vi "BK Precision 8600 Series Run List File.vi"() -> ()   [LabVIEW 2018]
doc: "Exemplifies how to run a stored list (sequence) from internal memory and measuring voltage and current while sequence is initiated."
uses:
  <instrlib>/BK Precision 8600 Series/BK Precision 8600 Series.lvlib
panel:
  in  "?":bool
  out "Current":dbl
  out "Voltage":dbl format="%_6f"
  in  "List Number (1)":i32=1 min=1 max=7 format="%#_0f"
  in  "VISA resource name":refnum<visa-resource-name>
  in  "Serial Configuration":cluster{"Baud Rate":u32}={"Baud Rate"=9600} {"Baud Rate" items=["300"=300, "600"=600, "1200"=1200, "2400"=2400, "4800"=4800, "9600"=9600, "19200"=19200]}
  # "(c) 2014-2019 B&K Precision Corporation.  ALL RIGHTS RESERVED."
  # "V"
  # "A"
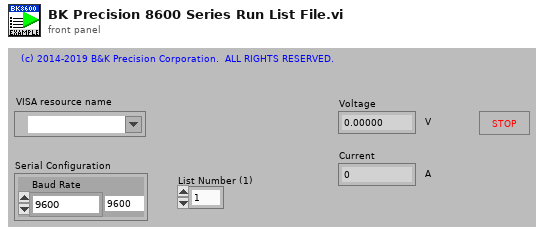
[diagram p1: front panel]
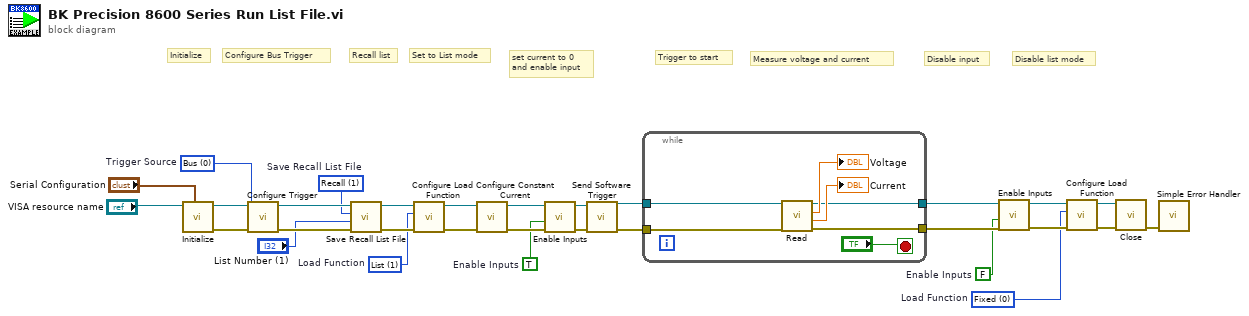
[diagram p0: block diagram]
diagram:
  w1 = u16 0 items=["Fixed", "List"]  # Load Function
  w3 = FALSE  # Enable Inputs
  w4 = TRUE  # Enable Inputs
  w2 = u16 1 items=["Fixed", "List"]  # Load Function
  w5 = u16 1 items=["Save", "Recall"]  # Save Recall List File
  w6 = u16 0 items=["Bus", "External", "Hold", "Manual", "Timed"]  # Trigger Source
  # "set current to 0\nand enable input"
  # "Measure voltage and current"
  # "Disable list mode"
  # "Set to List mode"
  # "Recall list"
  # "Configure Bus Trigger"
  # "Initialize"
  # "Trigger to start"
  # "Disable input"
  n1 = call <instrlib>:"Initialize.vi"("Serial Configuration"="Serial Configuration", "VISA resource name"="VISA resource name") -> ("error out"=w27:errorcluster, "VISA resource name out"=w28:refnum<visa-resource-name>)  [unwired: 8 in]
  n2 = call <instrlib>:"Configure Trigger.vi"("error in (no error)"=w27, "Trigger Source (0:Bus)"=w6, "VISA resource name"=w28) -> ("error out"=w24:errorcluster, "VISA resource name out"=w25:refnum<visa-resource-name>)  [unwired: 7 in]
  n3 = call <instrlib>:"Save Recall List File.vi"("error in (no error)"=w24, "List Number (1)"="List Number (1)", "Save Recall List File (0:Save)"=w5, "VISA resource name"=w25) -> ("error out"=w21:errorcluster, "VISA resource name out"=w22:refnum<visa-resource-name>)  [unwired: 6 in]
  n4 = call <instrlib>:"Configure Load Function.vi"("error in (no error)"=w21, "Load Function (0:Fixed)"=w2, "VISA resource name"=w22) -> ("error out"=w20:errorcluster, "VISA resource name out"=w19:refnum<visa-resource-name>)  [unwired: 7 in]
  n5 = call <instrlib>:"Configure Constant Current.vi"("error in (no error)"=w20, "VISA resource name"=w19) -> ("error out"=w18:errorcluster, "VISA resource name out"=w17:refnum<visa-resource-name>)  [unwired: 8 in]
  n6 = call <instrlib>:"Enable Inputs.vi"("error in (no error)"=w18, "Enable Input (F: False)"=w4, "VISA resource name"=w17) -> ("error out"=w15:errorcluster, "VISA resource name out"=w16:refnum<visa-resource-name>)  [unwired: 7 in]
  n7 = call <instrlib>:"Send Software Trigger.vi"("error in (no error)"=w15, "VISA resource name"=w16) -> ("error out"=w13:errorcluster, "VISA resource name out"=w14:refnum<visa-resource-name>)  [unwired: 8 in]
  n8 = while {
    tunnel: w14 -> [w35]
    tunnel: w13 -> [w34]
    tunnel: [w33] -> w12
    tunnel: [w32] -> w11
    stop <- "?" stop-if-true
    n9 = call <instrlib>:"Read.vi"("error in (no error)"=w34, "VISA resource name"=w35) -> ("error out"=w33:errorcluster, "Current"=→"Current":dbl, "Voltage"=→"Voltage":dbl, "VISA resource name out"=w32:refnum<visa-resource-name>)  [unwired: 6 in]
  }
  n10 = call <instrlib>:"Enable Inputs.vi"("error in (no error)"=w12, "Enable Input (F: False)"=w3, "VISA resource name"=w11) -> ("error out"=w9:errorcluster, "VISA resource name out"=w10:refnum<visa-resource-name>)  [unwired: 7 in]
  n11 = call <instrlib>:"Configure Load Function.vi"("error in (no error)"=w9, "Load Function (0:Fixed)"=w1, "VISA resource name"=w10) -> ("error out"=w7:errorcluster, "VISA resource name out"=w8:refnum<visa-resource-name>)  [unwired: 7 in]
  n12 = call <instrlib>:"Close.vi"("error in (no error)"=w7, "VISA resource name"=w8) -> ("error out"=w26:errorcluster)  [unwired: 9 in]
  n13 = call <vilib>:"Simple Error Handler.vi"("error in (no error)"=w26) -> ()  [unwired: 4 in, 5 out]
